vi "FEA_Model_Populate.vi"(3 "FEA_Model in":refnum<class "FEA_Model.lvclass">) -> (11 "FEA_Model out":refnum<class "FEA_Model.lvclass">)   [LabVIEW 2021, in "FEA_Model.lvclass"]
uses:
  FEA_Model.lvclass
  FEA_Model.lvclass/FEA_Model.ctl
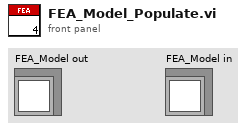
[diagram p1: front panel]
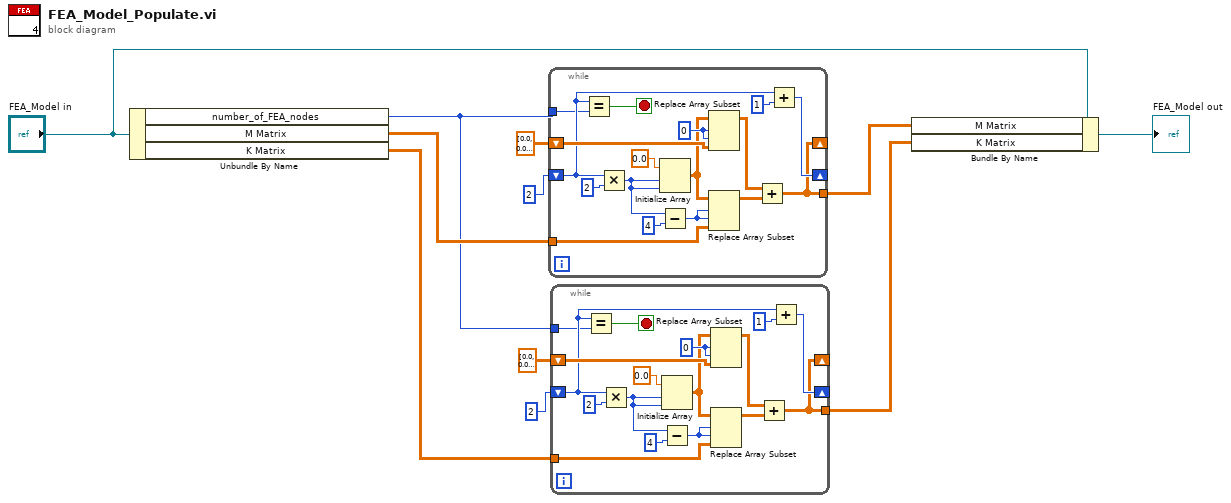
[diagram p0: block diagram]
diagram:
  n1 = Unbundle By Name("FEA_Model in") -> ("number_of_FEA_nodes"=w5:i32, "M Matrix"=w7:dbl[][], "K Matrix"=w6:dbl[][])
  n2 = while {
    shift-right: [w14] -> _
    shift-left: dbl[][] [[0.0, 0.0], [0.0, 0.0]] -> [w25]
    shift-right: [w21] -> _
    shift-left: 2 -> [w18]
    tunnel: w5 -> [w17]
    tunnel: w7 -> [w15]
    tunnel: [w14] -> w4
    stop <- w16 stop-if-true
    w24 = 0 ("index")
    n3 = Equal?(x=w18, y=w17) -> (x = y?=w16:bool)
    n4 = Multiply(x=w18, y=2) -> (x*y=w13:i32)
    n5 = Initialize Array(0.0 ("element"), w13, w13) -> (w12:dbl[][])
    n6 = Subtract(x=w13, y=4) -> (x-y=w23:i32)
    n7 = Replace Array Subset(array=w12, new element=w25, index (row)=w24, index (col)=w24) -> (w20:dbl[][])
    n8 = Replace Array Subset(array=w12, new element=w15, index (row)=w23, index (col)=w23) -> (w19:dbl[][])
    n9 = Add(x=w20, y=w19) -> (x+y=w14:dbl[][])
    n10 = Add(x=w18, y=1) -> (x+y=w21:i32)
  }
  n11 = while {
    shift-right: [w31] -> _
    shift-left: dbl[][] [[0.0, 0.0], [0.0, 0.0]] -> [w42]
    shift-right: [w38] -> _
    shift-left: 2 -> [w35]
    tunnel: w5 -> [w34]
    tunnel: w6 -> [w32]
    tunnel: [w31] -> w3
    stop <- w33 stop-if-true
    w41 = 0 ("index")
    n12 = Equal?(x=w35, y=w34) -> (x = y?=w33:bool)
    n13 = Multiply(x=w35, y=2) -> (x*y=w30:i32)
    n14 = Initialize Array(0.0 ("element"), w30, w30) -> (w29:dbl[][])
    n15 = Subtract(x=w30, y=4) -> (x-y=w40:i32)
    n16 = Replace Array Subset(array=w29, new element=w42, index (row)=w41, index (col)=w41) -> (w37:dbl[][])
    n17 = Replace Array Subset(array=w29, new element=w32, index (row)=w40, index (col)=w40) -> (w36:dbl[][])
    n18 = Add(x=w37, y=w36) -> (x+y=w31:dbl[][])
    n19 = Add(x=w35, y=1) -> (x+y=w38:i32)
  }
  n20 = Bundle By Name(cluster="FEA_Model in", "M Matrix"=w4, "K Matrix"=w3) -> (→"FEA_Model out":refnum<class "FEA_Model.lvclass">)
